vi "MotorMultiSelect.vi"(3 "Motor":string[](array[string]), 9 "error in (no error)":errorcluster) -> (0 "Motor out":string[](array[string]), 6 "error out":errorcluster)   [LabVIEW 2009]
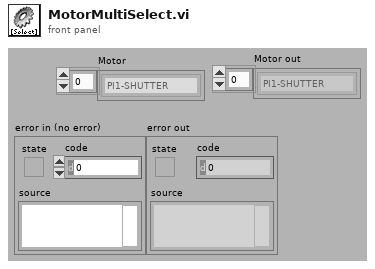
[diagram p1: front panel]
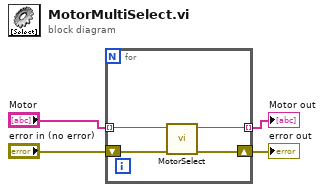
[diagram p0: block diagram]
diagram:
  n1 = for {
    tunnel: "Motor" -> [w6] mode=indexing
    shift-right: [w7] -> w2
    shift-left: "error in (no error)" -> [w8]
    tunnel: [w5] -> w1 mode=indexing
    n2 = call "MotorSelect.vi"("Motor"=w6, "error in (no error)"=w8) -> ("Motor out"=w5:string, "error out"=w7:errorcluster)  [unwired: 6 out]
  }
  "error out" <- w2
  "Motor out" <- w1
